vi "correlation.vi"(0 "X":cdb[](array[numeric]), 3 "Y":cdb[](array[numeric])) -> (7 "Correlation":cdb[](array[numeric]))   [LabVIEW 2012]
uses:
  <vilib>/Analysis/NI_AALPro.lvlib
panel:
  out "subarray":cdb[](array[numeric])
  out "Shifted Array":dbl[][](array[numeric])
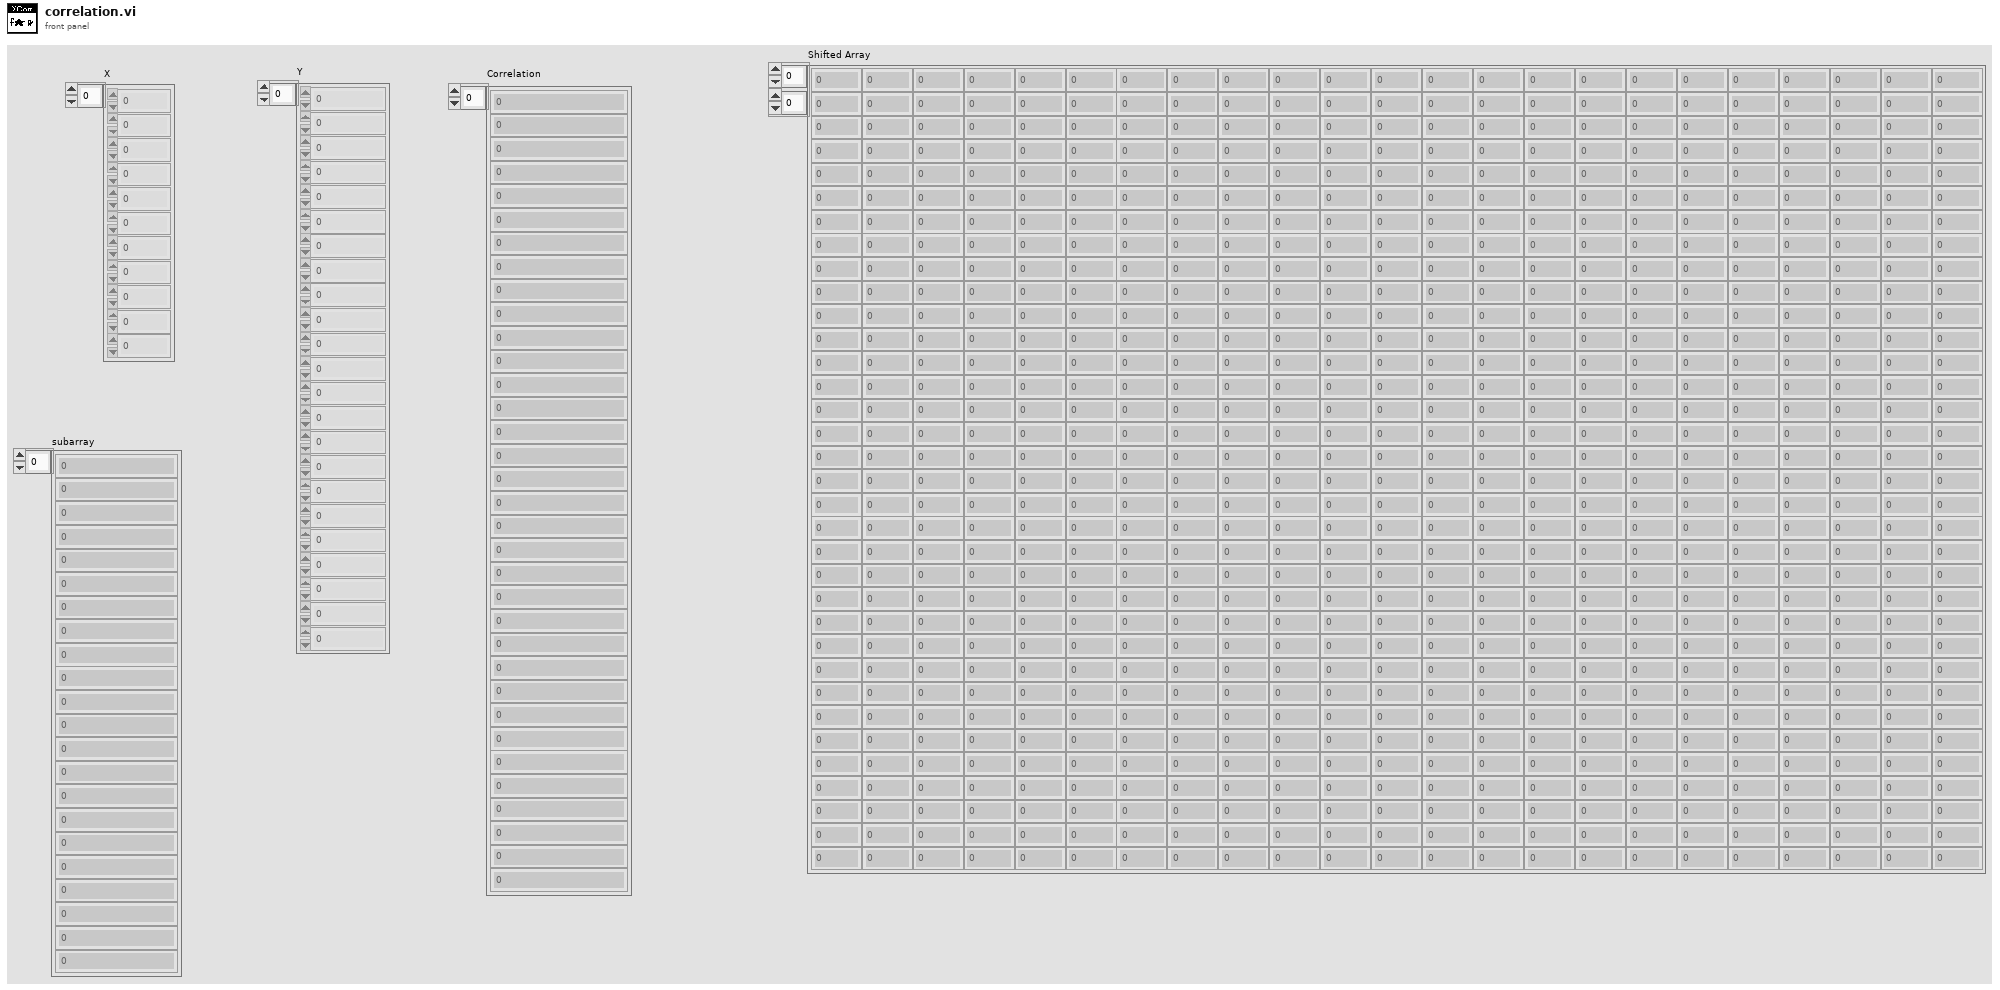
[diagram p1: front panel]
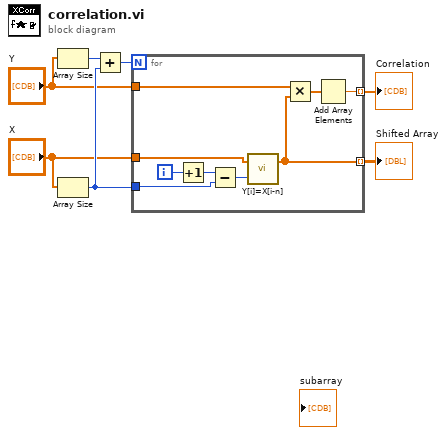
[diagram p0: block diagram]
diagram:
  n1 = Array Size(array="Y") -> (size(s)=w5:i32)
  n2 = Array Size(array="X") -> (size(s)=w4:i32)
  n3 = Add(x=w5, y=w4) -> (x+y=w3:i32)
  n4 = for {
    N: w3 -> [_]
    tunnel: "Y" -> [w15]
    tunnel: "X" -> [w16]
    tunnel: [w13] -> w7 mode=indexing
    tunnel: w4 -> [w12]
    tunnel: [w10] -> w6 mode=indexing
    i -> [w9]
    n5 = Increment(x=w9) -> (x+1=w8:i32)
    n6 = Subtract(x=w8, y=w12) -> (x-y=w11:i32)
    n7 = call <vilib>:"Y[i]=X[i-n].vi"("shifts: n"=w11, "Input Array"=w16) -> ("Shifted Array"=w10:dbl[])  [unwired: 1 out]
    n8 = Multiply(x=w15, y=w10) -> (x*y=w14:cdb[])
    n9 = Add Array Elements(numeric array=w14) -> (sum=w13:cdb)
  }
  "Correlation" <- w7
  "Shifted Array" <- w6
